vi "2D Cartesian Coordinate Shift.vi"   [LabVIEW 2024, in "NI_AALPro.lvlib"]
doc: "<p>Shifts two-dimensional Cartesian coordinates along the x- and y-axes. Wire data to the <strong>X</strong> input to determine the polymorphic instance to use or <a href=\"nihelplauncher://docs/csh?context=lvcore_lvhowto_selectingdefaultinstpolyvi\">manually select</a> the instance.\n</p>"
uses:
  NI_AALPro.lvlib
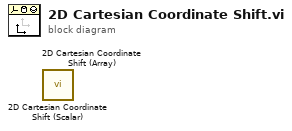
[diagram p0: block diagram]
diagram:
  n1 = call "2D Cartesian Coordinate Shift (Scalar).vi"() -> ()  [unwired: 9 in, 3 out]
  n2 = call "2D Cartesian Coordinate Shift (Array).vi"() -> ()  [unwired: 9 in, 3 out]
